vi "FIRE_routine.vi"(11 "StateIn":dbl) -> (3 "StateOut":dbl)   [LabVIEW 2012]
uses:
  <vilib>/Rock Robotics/WPI/Solenoid/WPI_SolenoidValue.ctl
  Autonomous_Routine_Global.vi
  <vilib>/Rock Robotics/WPI/Solenoid/WPI_SolenoidSetEnum.vi
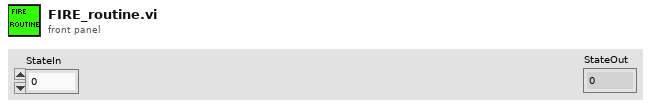
[diagram p1: front panel]
types:
  T1 = typedef "WPI_SolenoidValue.ctl" = enum16{"Off", "On", "Forward", "Reverse"}
  T2 = typedef "WPI_AnalogChannelDevRef.ctl" = cluster{"DevStatus":errorcluster, "Analog Module":T3, "Analog Channel":T4}
  T3 = typedef "FPGA_TypedefAnalogModule.ctl" = enum16{"Analog Module 1", "Analog Module 2"}
  T4 = typedef "FPGA_AIChannel.ctl" = enum8{"AI 1", "AI 2", "AI 3", "AI 4", "AI 5", "AI 6", "AI 7", "AI 8", "Invalid"}
  T5 = typedef "WPI_SolenoidDevRef.ctl" = cluster{"DevStatus":errorcluster, "Solenoid Module":T6, "Forward Solenoid Channel":T7, "Reverse Solenoid Channel":T7}
  T6 = typedef "FPGA_TypedefSolenoidModule.ctl" = enum16{"Solenoid Module 1", "Solenoid Module 2"}
  T7 = typedef "WPI_SolenoidChannel.ctl" = enum8{"Solenoid 1", "Solenoid 2", "Solenoid 3", "Solenoid 4", "Solenoid 5", "Solenoid 6", "Solenoid 7", "Solenoid 8", "Invalid"}
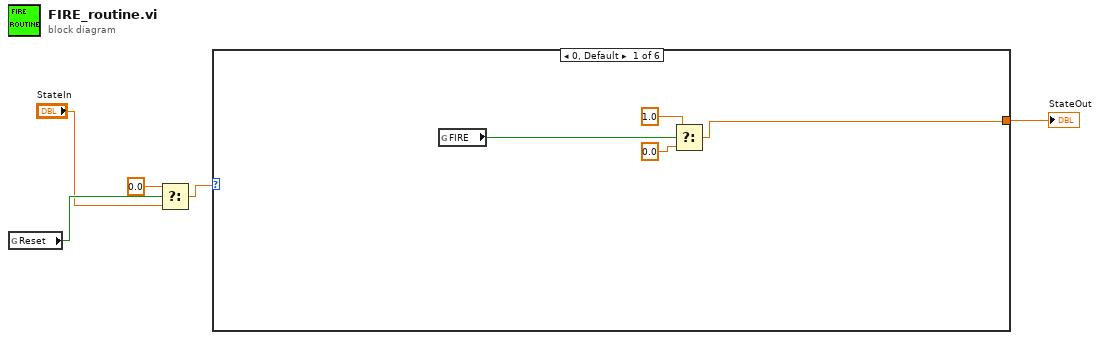
[diagram p0: block diagram]
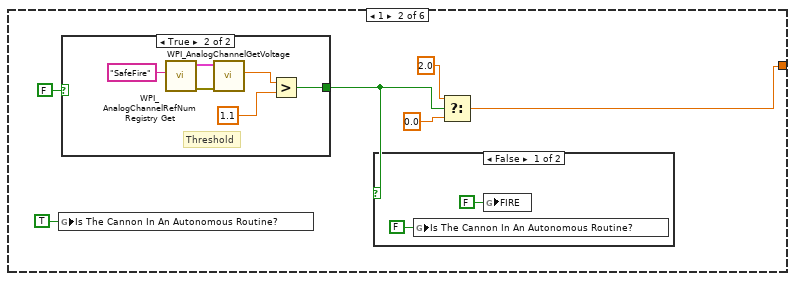
[diagram p2: hidden frame]
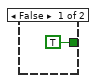
[diagram p4: hidden frame]
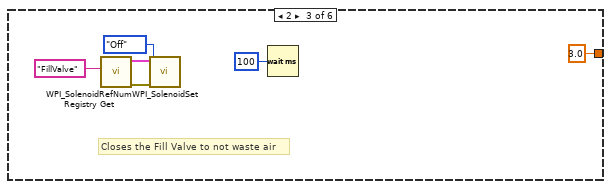
[diagram p5: hidden frame]
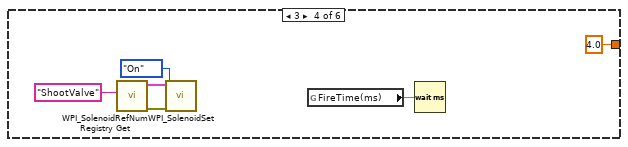
[diagram p6: hidden frame]
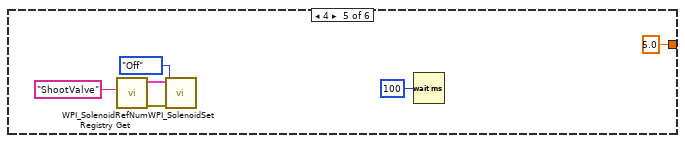
[diagram p7: hidden frame]
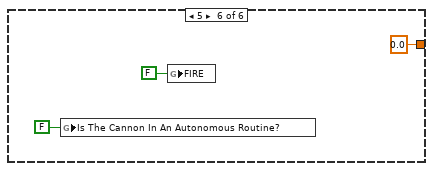
[diagram p8: hidden frame]
diagram:
  n1 = global read "Autonomous_Routine_Global.vi" "Reset"() -> (w3:bool)
  n2 = Select(t=0.0, s=w3, f="StateIn") -> (s? t:f=w4:dbl)
  n3 = case shown="0, Default" w4 {
    tunnel: [w6 w10 3.0 ("f") 4.0 ("f") 5.0 ("f") 0.0 ("f")] -> w5
    frame 0, Default {
      n4 = global read "Autonomous_Routine_Global.vi" "FIRE"() -> (w9:bool)
      n5 = Select(t=1.0, s=w9, f=0.0) -> (s? t:f=w6:dbl)
    }
    frame 1 {
      n6 = global write "Autonomous_Routine_Global.vi" "Is The Cannon In An Autonomous Routine?"(TRUE ("Is The Cannon In An Autonomous Routine?")) -> ()
      n7 = case shown="True" FALSE {
        tunnel: [TRUE w19] -> w12
        frame False {
        }
        frame True {
          # "Threshold"
          n8 = call <vilib>:"WPI_AnalogChannelRefNum Registry Get.vi"("refnum name"="SafeFire") -> ("error out"=w23:errorcluster, "AIDeviceRef"=w22:T2)  [unwired: 9 in]
          n9 = call <vilib>:"WPI_AnalogChannelGetVoltage.vi"("error in (no error)"=w23, "AIDeviceRef"=w22) -> ("Voltage"=w21:dbl)  [unwired: 7 in, 2 out]
          n10 = Greater?(x=w21, y=1.1) -> (0:w19:bool)
        }
      }
      n11 = case shown="False" w12 {
        frame False {
          n12 = global write "Autonomous_Routine_Global.vi" "Is The Cannon In An Autonomous Routine?"(FALSE ("Is The Cannon In An Autonomous Routine?")) -> ()
          n13 = global write "Autonomous_Routine_Global.vi" "FIRE"(FALSE ("FIRE")) -> ()
        }
        frame True {
        }
      }
      n14 = Select(t=2.0, s=w12, f=0.0) -> (s? t:f=w10:dbl)
    }
    frame 2 {
      # "Closes the Fill Valve to not waste air"
      n15 = call <vilib>:"WPI_SolenoidRefNum Registry Get.vi"("refnum name"="FillValve") -> ("error out"=w30:errorcluster, "SolenoidDevRef"=w29:T5)  [unwired: 9 in]
      n16 = call-poly <vilib>:"WPI_SolenoidSet.vi"("error in (no error)"=w30, "Value"=WPI_SolenoidValue."Off", "SolenoidDevRef"=w29) -> ()  [unwired: 7 in, 2 out]
      n17 = Wait (ms)(milliseconds to wait=u32 100) -> ()  [unwired: 1 out]
    }
    frame 3 {
      n18 = call <vilib>:"WPI_SolenoidRefNum Registry Get.vi"("refnum name"="ShootValve") -> ("error out"=w33:errorcluster, "SolenoidDevRef"=w34:T5)  [unwired: 9 in]
      n19 = call-poly <vilib>:"WPI_SolenoidSet.vi"("error in (no error)"=w33, "Value"=WPI_SolenoidValue."On", "SolenoidDevRef"=w34) -> ()  [unwired: 7 in, 2 out]
      n20 = global read "Autonomous_Routine_Global.vi" "FireTime(ms)"() -> (w32:dbl)
      n21 = Wait (ms)(milliseconds to wait=w32) -> ()  [unwired: 1 out]
    }
    frame 4 {
      n22 = call <vilib>:"WPI_SolenoidRefNum Registry Get.vi"("refnum name"="ShootValve") -> ("error out"=w42:errorcluster, "SolenoidDevRef"=w41:T5)  [unwired: 9 in]
      n23 = call-poly <vilib>:"WPI_SolenoidSet.vi"("error in (no error)"=w42, "Value"=WPI_SolenoidValue."Off", "SolenoidDevRef"=w41) -> ()  [unwired: 7 in, 2 out]
      n24 = Wait (ms)(milliseconds to wait=u32 100) -> ()  [unwired: 1 out]
    }
    frame 5 {
      n25 = global write "Autonomous_Routine_Global.vi" "Is The Cannon In An Autonomous Routine?"(FALSE ("FIRE")) -> ()
      n26 = global write "Autonomous_Routine_Global.vi" "FIRE"(FALSE ("FIRE")) -> ()
    }
  }
  "StateOut" <- w5
